vi "Action Set Fault.vi"(5 "Retry Attempts (0)":i32 min=0, 8 "error in":errorcluster, 11 "VISA resource name":refnum<visa-resource-name>) -> (0 "error out":errorcluster, 3 "VISA resource name out":refnum<visa-resource-name>)   [LabVIEW 2020, in "ChromTech Series III Pump.lvlib"]
doc: "Stop the pump."
uses:
  ChromTech Series III Pump.lvlib
panel:
  out "Response":string
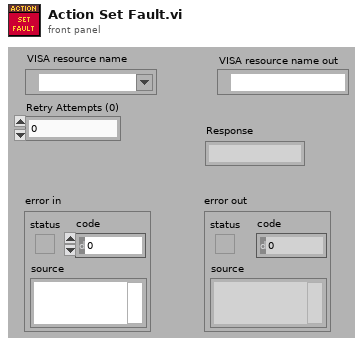
[diagram p1: front panel]
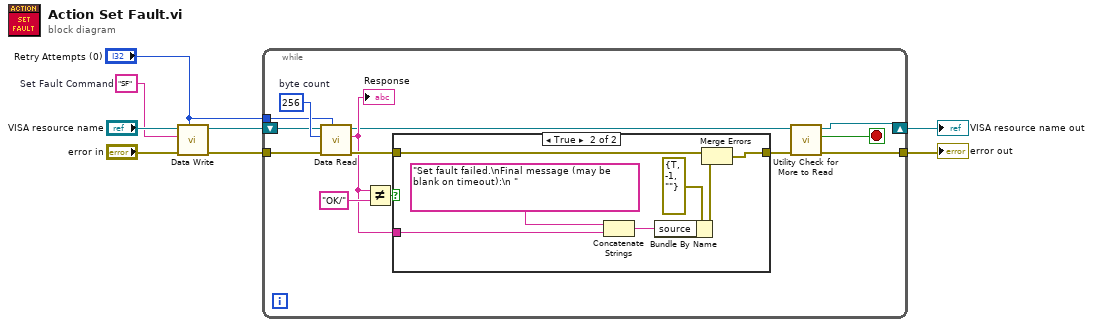
[diagram p0: block diagram]
diagram:
  w6 = "SF"  # Set Fault Command
  n1 = call "Data Write.vi"("Retry Attempts (0)"="Retry Attempts (0)", "error in (no error)"="error in", "Command"=w6, "VISA Refnum in"="VISA resource name") -> ("error out"=w5:errorcluster, "VISA Refnum out"=w4:refnum<visa-resource-name>)  [unwired: 6 in]
  n2 = while {
    shift-right: [w11] -> w2
    shift-left: w4 -> [w16]
    tunnel: "Retry Attempts (0)" -> [w10]
    tunnel: w5 -> [w17]
    tunnel: [w13] -> w3
    stop <- w9 stop-if-true
    w21 = u32 256  # byte count
    n3 = call "Data Read.vi"("Retry Attempts (0)"=w10, "error in (no error)"=w17, "Bytes to read"=w21, "VISA Refnum in"=w16) -> ("error out"=w18:errorcluster, "read buffer"=w15:string, "VISA Refnum out"=w12:refnum<visa-resource-name>)  [unwired: 5 in]
    "Response" <- w15
    n4 = Not Equal?(x=w15, y="OK/") -> (x != y?=w19:bool)
    n5 = case shown="True" w19 {
      tunnel: [w22 w28] -> w14
      tunnel: w18 -> [w22 w27]
      tunnel: w15 -> [_ w23]
      frame False {
      }
      frame True {
        n6 = Concatenate Strings("Set fault failed.\nFinal message (may be blank on timeout):\n ", w23) -> (w25:string)
        n7 = Bundle By Name(cluster=errorcluster {"status"=TRUE, "code"=-1, "source"=""} ("error out"), "source"=w25) -> (w26:errorcluster)
        n8 = Merge Errors(w27, w26) -> (w28:errorcluster)
      }
    }
    n9 = call "Utility Check for More to Read.vi"("error in (no error)"=w14, "VISA Refnum in"=w12) -> ("error out (unchanged)"=w13:errorcluster, "More to read?"=w9:bool, "VISA Refnum out"=w11:refnum<visa-resource-name>)  [unwired: 7 in]
  }
  "VISA resource name out" <- w2
  "error out" <- w3
